vi "Close References.vi"(8 "error in (no error)":errorcluster, 11 "motor communication in":refnum<class "NI_Robotics_Motor Communication Ref.lvclass">) -> (0 "error out":errorcluster)   [LabVIEW 2017, in "NI_Robotics_Motor Communication Ref.lvclass"]
uses:
  <vilib>/robotics/Actuation/Motor Communication Ref/NI_Robotics_Motor Communication Ref.lvclass
  c:/Program Files (x86)/National Instruments/LabVIEW 2017/vi.lib/robotics/Actuation/Motor Communication/NI_Robotics_Motor Communication.lvclass
  <vilib>/robotics/Actuation/Motor Communication Ref/NI_Robotics_Motor Communication Ref.lvclass/NI_Robotics_Motor Communication Ref.ctl
  <vilib>/robotics/Actuation/Motor Communication/NI_Robotics_Motor Communication.lvclass/NI_Robotics_Motor Communication.ctl
  <vilib>/robotics/Actuation/Motor Communication Ref/FG Motor Comm Ref Sessions Action.ctl
  <vilib>/robotics/Actuation/Motor Communication/NI_Robotics_Motor Communication.lvclass
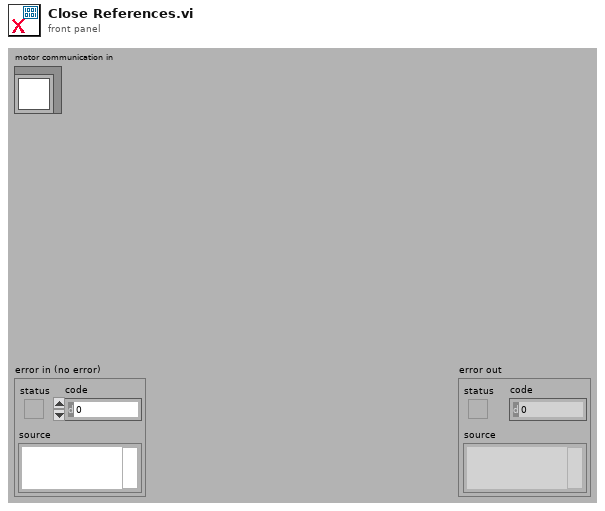
[diagram p1: front panel]
types:
  T1 = typedef "NI_Robotics_Motor Communication Ref.lvclass/FG Motor Comm Ref Sessions Action.ctl" = enum16{"Get", "Add", "Delete"}
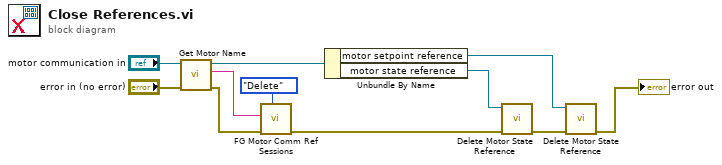
[diagram p0: block diagram]
diagram:
  n1 = call <vilib>:"Get Motor Name.vi"("error in (no error)"="error in (no error)", "motor communication in"="motor communication in") -> ("error out"=w7:errorcluster, "motor name"=w9:string, "motor communication out"=w6:refnum<class "NI_Robotics_Motor Communication Ref.lvclass">)  [unwired: 7 in]
  n2 = call <vilib>:"FG Motor Comm Ref Sessions.vi"("action"=FG_Motor_Comm_Ref_Sessions_Action."Delete", "error in (no error)"=w7, "motor name"=w9) -> ("error out"=w4:errorcluster)  [unwired: 6 in, 2 out]
  n3 = Unbundle By Name(w6) -> ("motor setpoint reference"=w2:refnum<data-value>, "motor state reference"=w5:refnum<data-value>)
  n4 = call <vilib>:"Delete Motor State Reference.vi"("error in (no error)"=w4, "motor state ref"=w5) -> ("error out"=w3:errorcluster)  [unwired: 9 in]
  n5 = call <vilib>:"Delete Motor State Reference.vi"("error in (no error)"=w3, "motor state ref"=w2) -> ("error out"=→"error out":errorcluster)  [unwired: 9 in]
